vi "instance count allowed.vi"(8 "error in":errorcluster, 11 "fixed module parent implementation configuration in":refnum<class "fixed channel configuration.lvclass">) -> (0 "error out":errorcluster, 2 "instances allowed":i32, 3 "fixed module parent implementation configuration out":refnum<class "fixed channel configuration.lvclass">)   [LabVIEW 2013, in "fixed channel configuration.lvclass"]
uses:
  fixed channel configuration.lvclass
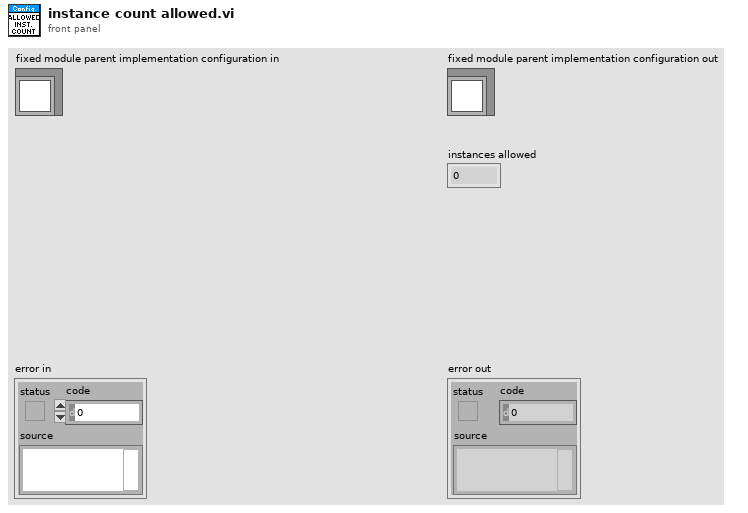
[diagram p1: front panel]
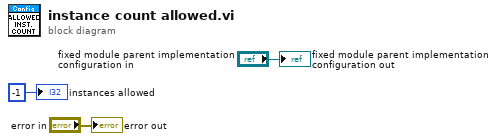
[diagram p0: block diagram]
diagram:
  "error out" <- "error in"
  "fixed module parent implementation configuration out" <- "fixed module parent implementation configuration in"
  "instances allowed" <- -1 ("instances allowed")
